vi "LiftManualSelectHeight.vi"() -> ()   [LabVIEW 2014, in "LiftLib.lvlib"]
uses:
  LiftLib.lvlib
panel:
  in  "Height":dbl
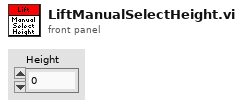
[diagram p1: front panel]
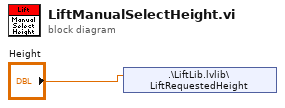
[diagram p0: block diagram]
diagram:
  n1 = shared-variable ".\\LiftLib.lvlib\\LiftRequestedHeight"("Height") -> ()  [unwired: 1 in, 1 out]
